vi "DB_set_and_save.vi"(6 "database_inf":T2, 7 "New Date Name":string, 8 "error in (no error)":errorcluster, 9 "Value":T1[](array[typedef]), 10 "Chemical":string="Xenon", 11 "Scan Type":string="Xenon") -> (0 "error out":errorcluster)   [LabVIEW 2019]
uses:
  Type defs/data_cred.ctl
  Type defs/cred_ip_info.ctl
  lv_mysql_connector_v1_lv8/typedefs/mysql_authentication.ctl
  Type defs/FileAcq_v1_Ctrl.ctl
  Ctrl/FileAcq_v1_Ctrl.ctl
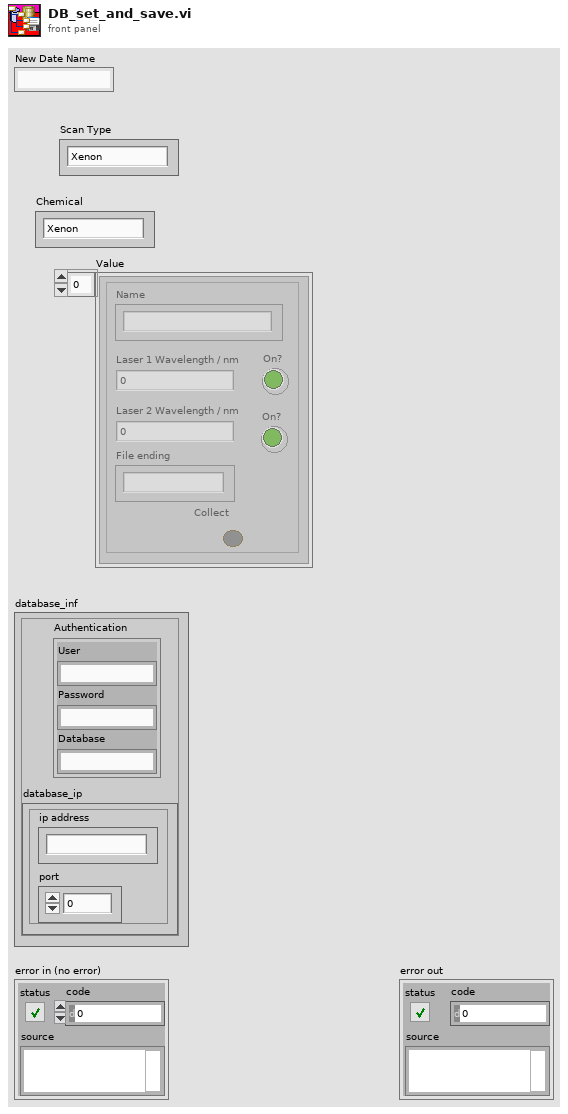
[diagram p1: front panel]
types:
  T1 = typedef "FileAcq_v1_Ctrl.ctl" = cluster{"Type":string, "LaserWave1":dbl, "Shutter1":bool, "LaserWave2":dbl, "Shutter2":bool, "FileEnd":string, "Collect":bool}
  T2 = typedef "data_cred.ctl" = cluster{"database_ip":T3, "Authentication":T4}
  T3 = typedef "cred_ip_info.ctl" = cluster{"ip address":string, "port":dbl}
  T4 = typedef "mysql_authentication.ctl" = cluster{"User":string, "Password":string, "Database":string}
  T5 = typedef "Database_control.ctl" = cluster{"filename":string, "date":string, "type":string, "chemical":string, "experiment":string, "laser1":dbl, "laser2":dbl}
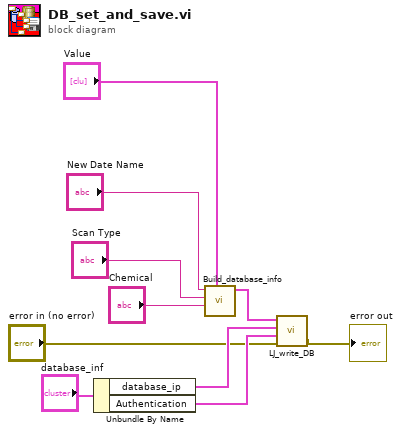
[diagram p0: block diagram]
diagram:
  n1 = Unbundle By Name("database_inf") -> ("database_ip"=w9:T3, "Authentication"=w10:T4)
  n2 = call "Build_database_info.vi"("Collection Info Array"="Value", "Chemical"="Chemical", "RingText.Text"="Scan Type", "New Date Name"="New Date Name") -> ("Data to add"=w7:T5)  [unwired: 7 in]
  n3 = call "LJ_write_DB.vi"("error in"="error in (no error)", "Authentication"=w10, "database_ip"=w9, "Data to add"=w7) -> ("error out"=→"error out":errorcluster)  [unwired: 1 in]
